vi "Create Digital Waveform.vi"() -> ()   [LabVIEW 2023]
doc: "This example illustrates how the use of the Digital Data controls and how to construct a Digital Waveform from individual components. A Digital Waveform Graph represents the signals graphically. Attention is placed on the distinctions of signal versus sample and directions are given on displaying the plots in the form of a single bus or individually."
panel:
  in  "Digital Data":digitaldata={"transitions"=[], "data"=[[0, 0, 0, 0, 0, 0, 1, 0], [0, 0, 0, 0, 0, 1, 1, 1], [0, 0, 0, 0, 0, 1, 0, 0], [0, 0, 1, 0, 1, 1, 0, 1], [1, 1, 1, 1, 1, 1, 1, 1]]}
  out "Digital Waveform Graph":digitalwaveform(graph)
  # "Overview: Creates a digital waveform from the specified digital data.\nInstructions:\nRun the VI."
  # "Each column within Digital Data is a signal that appears as a row in the Digital Waveform Graph. Each row is a sample. To see the numerical value of a given sample, right-click one of the signal values on the Y Axis and deselect Expand Digital Buses."
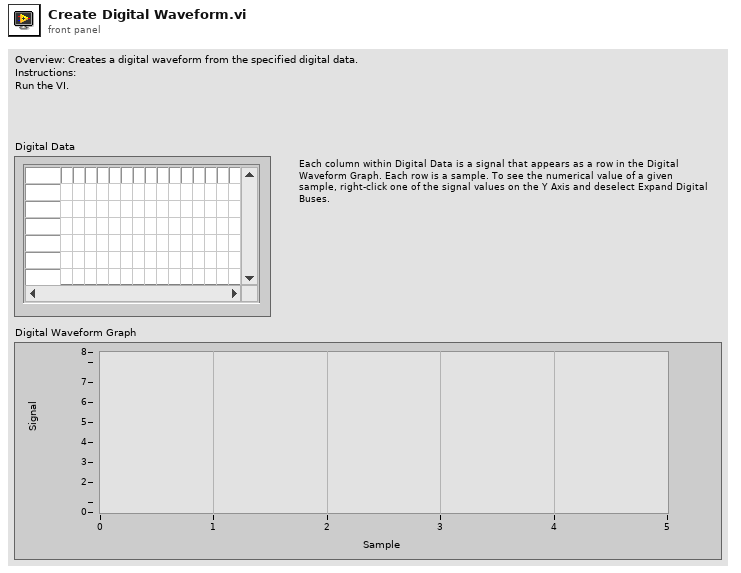
[diagram p1: front panel]
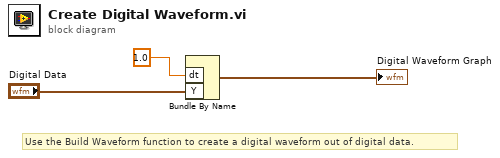
[diagram p0: block diagram]
diagram:
  # "Use the Build Waveform function to create a digital waveform out of digital data."
  n1 = Bundle By Name("dt"=1.0, "Y"="Digital Data") -> (→"Digital Waveform Graph":digitalwaveform)  [unwired: 1 in]
